vi "Add Client to Service.vi"(8 "error in (no error)":errorcluster, 9 "Client ID":string, 10 "WebSocket Connection in":refnum<k5>, 11 "WebSocket Server in":refnum<class "WebSocket Server.lvclass">) -> (0 "error out":errorcluster, 3 "WebSocket Server out":refnum<class "WebSocket Server.lvclass">)   [LabVIEW 2016, in "WebSocket Actors.lvlib" / "WebSocket Server.lvclass"]
uses:
  WebSocket Server.lvclass
  WebSocket Server.lvclass/WebSocket Server.ctl
  <vilib>/GPower/Error/Library/SplitAppended.vi
  <vilib>/GPower/Error/Library/AppendErrors.vi
  <vilib>/GPower/Error/Library/Append/AppendMulti.vi
  <vilib>/GPower/Error/Library/SubVIs/ExplanationToError.vi
  <vilib>/dlg_ctls.llb/Space Constant.vi
  <vilib>/Utility/error.llb/Trim Whitespace.vi
  <vilib>/Utility/error.llb/Error Code Database.vi
  <vilib>/GPower/Error/Library/Append/AppendSingle.vi
  WebSocket Service Messages/Add Client Msg/Add Client Msg.lvclass
  WebSockets/WebSockets.lvlib
  <vilib>/GPower/Error/GPError.lvlib
panel:
  out "Resource Name":string
  out "HTTP Headers":variant
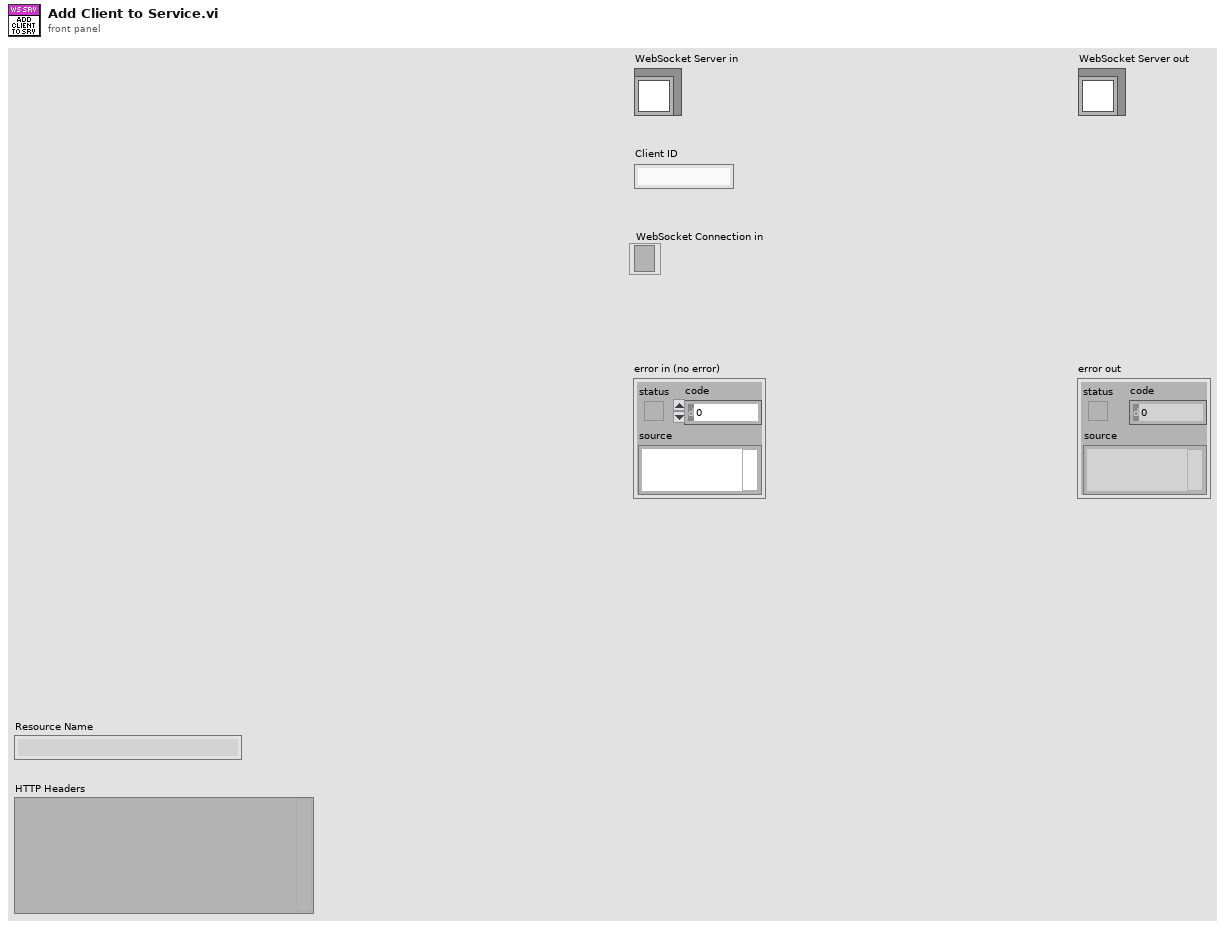
[diagram p1: front panel]
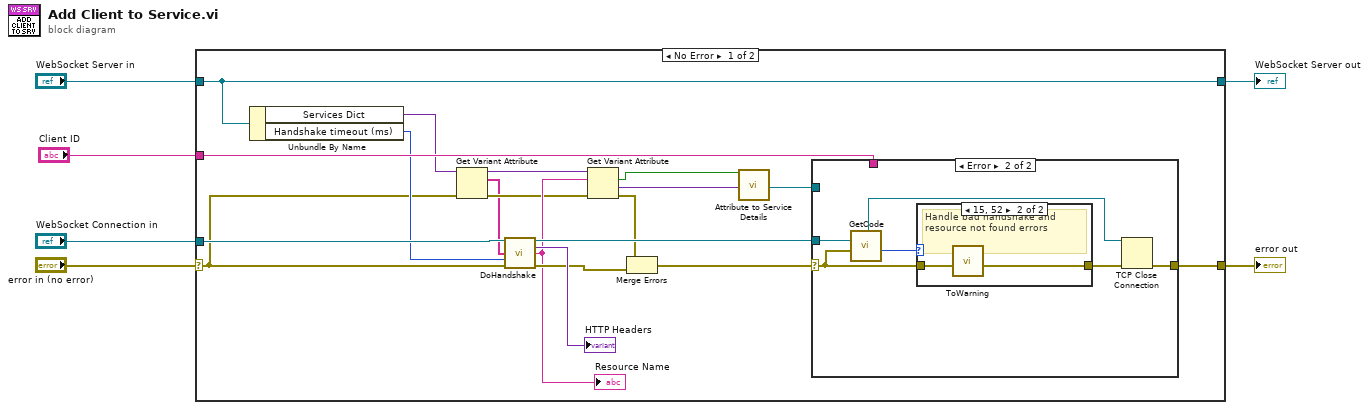
[diagram p0: block diagram]
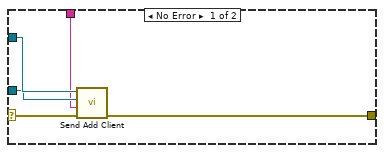
[diagram p2: hidden frame]
diagram:
  n1 = case shown="No Error" "error in (no error)" {
    selector: "error in (no error)" -> [w10 w40]
    tunnel: [w15 w40] -> w5
    tunnel: [w21 w39] -> w3
    tunnel: "WebSocket Server in" -> [w21 w39]
    tunnel: "WebSocket Connection in" -> [w22 _]
    tunnel: "Client ID" -> [w14 _]
    frame No Error {
      n2 = Unbundle By Name(w21) -> ("Services Dict"=w11:variant, "Handshake timeout (ms)"=w12:i32)
      n3 = Get Variant Attribute(Variant=w11, error in=w10) -> (duplicate Variant=w8:variant, names=w7:string[], error out=w9:errorcluster)  [unwired: 2 in, 1 out]
      n4 = call "DoHandshake.vi"("WebSocket Connection in"=w22, "Resource Names"=w7, "timeout ms (5000)"=w12, "error in (no error)"=w10) -> ("WebSocket Connection out"=w24:refnum<k5>, "Headers Out"=→"HTTP Headers":variant, "Resource Name"=w13:string, "error out"=w20:errorcluster)  [unwired: 6 in, 2 out]
      "Resource Name" <- w13
      n5 = Get Variant Attribute(Variant=w8, name=w13, error in=w9) -> (found=w18:bool, value=w17:variant, error out=w19:errorcluster)  [unwired: 1 in, 1 out]
      n6 = Merge Errors(w19, w20) -> (w23:errorcluster)
      n7 = call "Attribute to Service Details.vi"("Attibute Found"=w18, "Attribute"=w17) -> ("Service Enqueuer"=w16:refnum<class "Message Enqueuer.lvclass">)  [unwired: 17 in]
      n8 = case shown="Error" w23 {
        selector: w23 -> [w30 w32]
        tunnel: w24 -> [w27 w34]
        tunnel: [w29 w35] -> w15
        tunnel: w16 -> [w28 _]
        tunnel: w14 -> [w26 _]
        frame No Error {
          n9 = call "Send Add Client.vi"("error in (no error)"=w30, "Client ID"=w26, "WebSocket Connection"=w27, "Message Enqueuer in"=w28) -> ("error out"=w29:errorcluster)  [unwired: 6 in, 1 out]
        }
        frame Error {
          n10 = call <vilib>:"GetCode.vi"("Error in"=w32) -> ("Code"=w33:i32)  [unwired: 10 in]
          n11 = case shown="15, 52" w33 {
            tunnel: w32 -> [w36 w38]
            tunnel: [w36 w37] -> w31
            frame 0, Default {
              # "Unknown error"
            }
            frame 15, 52 {
              # "Handle bad handshake and resource not found errors"
              n12 = call <vilib>:"ToWarning.vi"("Error in"=w38) -> ("Warning out"=w37:errorcluster)  [unwired: 10 in]
            }
          }
          n13 = TCP Close Connection(connection ID=w34, error in (no error)=w31) -> (error out=w35:errorcluster)  [unwired: 1 in, 1 out]
        }
      }
    }
    frame Error {
    }
  }
  "error out" <- w5
  "WebSocket Server out" <- w3
